vi "statsCalcWithWrite.vi"() -> ()   [LabVIEW 2014]
uses:
  <vilib>/gmath/statdist.llb/Normal Random.vi
  <userlib>/StatsCalculatorLabView/StatsCalculatorLabView.lvlib
  <vilib>/gmath/NI_Gmath.lvlib
  <vilib>/Analysis/NI_AALBase.lvlib
panel:
  in  "Output\nFilename":string="statsSummary.txt"
  out "VI Name":string
  out "Gaussian Distribution":T1(graph)
  out "Error State":errorcluster
  out "Standard Deviation":dbl(knob) scale=0.0..10.0
  out "Mean":dbl(knob) scale=0.0..10.0
  out "Sum":dbl(knob) scale=0.0..10.0
  in  "True\nStandard Deviation":dbl(knob)=0.5 scale=0.5..2.0
  in  "True Mean":dbl(knob) scale=-5.0..5.0
  in  "Number of Values":i32(knob)=50 scale=100.0..1000.0
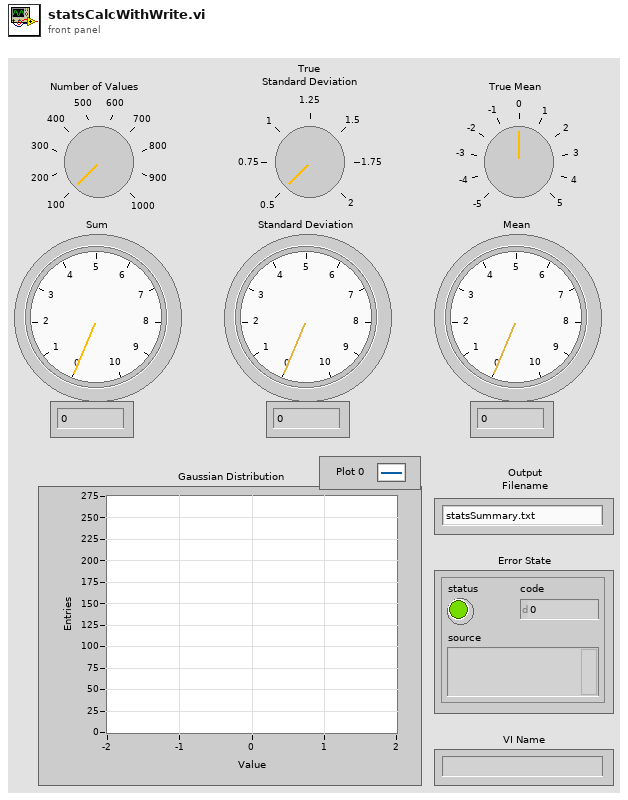
[diagram p1: front panel]
types:
  T1 = cluster{"X Values":dbl[], "Histogram: h(x)":i32[]}
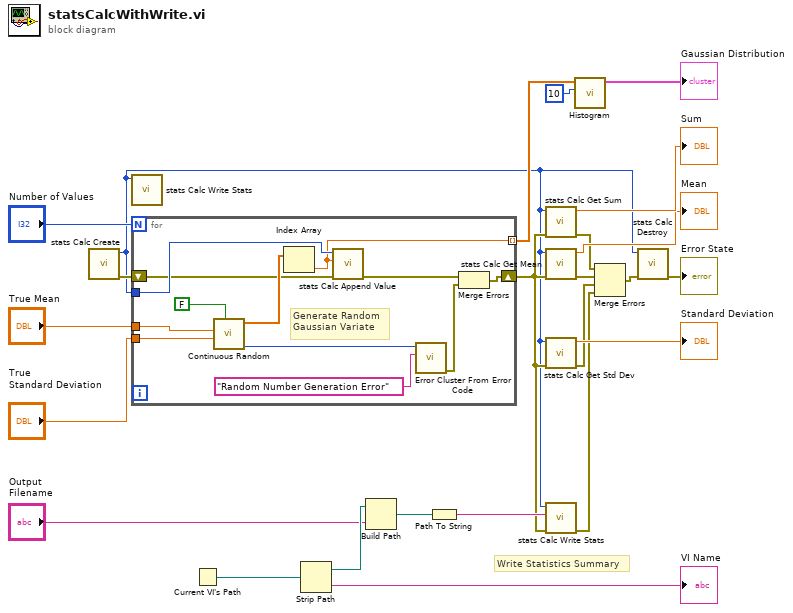
[diagram p0: block diagram]
diagram:
  # "Write Statistics Summary"
  n1 = call <userlib>:"stats Calc Create.vi"() -> ("error out"=w21:errorcluster, "function return"=w2:i32)  [unwired: 10 in]
  n2 = call <userlib>:"stats Calc Write Stats.vi"("handle"=w2) -> ()  [unwired: 10 in, 1 out]
  n3 = for {
    N: "Number of Values" -> [_]
    tunnel: w2 -> [w36]
    tunnel: "True\nStandard Deviation" -> [w35]
    tunnel: "True Mean" -> [w34]
    shift-right: [w26] -> w3
    shift-left: w21 -> [w29]
    tunnel: [w25] -> w12 mode=indexing
    # "Generate Random\nGaussian Variate"
    n4 = call-poly <vilib>:"Continuous Random.vi"("reset"=FALSE, "std"=w35, "mean"=w34) -> ("error"=w31:i32, "normal random data"=w32:dbl[])  [unwired: 7 in]
    n5 = Index Array(array=w32) -> (element=w25:dbl)  [unwired: 1 in]
    n6 = call <userlib>:"stats Calc Append Value.vi"("error in (no error)"=w29, "value"=w25, "handle"=w36) -> ("error out"=w27:errorcluster)  [unwired: 8 in]
    n7 = call <vilib>:"Error Cluster From Error Code.vi"("error message (\"\")"="Random Number Generation Error", "error code (0)"=w31) -> ("error out"=w28:errorcluster)  [unwired: 7 in]
    n8 = Merge Errors(w27, w28) -> (w26:errorcluster)
  }
  n9 = Current VI's Path() -> (path=w9:path)
  n10 = Strip Path(path=w9) -> (stripped path=w7:path, name=→"VI Name":string)
  n11 = Build Path(base path=w7, name or relative path="Output\nFilename") -> (appended path=w5:path)
  n12 = Path To String(path=w5) -> (string=w4:string)
  n13 = call <userlib>:"stats Calc Get Sum.vi"("error in (no error)"=w3, "handle"=w2) -> ("error out"=w17:errorcluster, "function return"=→"Sum":dbl)  [unwired: 8 in]
  n14 = call <userlib>:"stats Calc Get Mean.vi"("error in (no error)"=w3, "handle"=w2) -> ("error out"=w16:errorcluster, "function return"=→"Mean":dbl)  [unwired: 8 in]
  n15 = call <userlib>:"stats Calc Get Std Dev.vi"("error in (no error)"=w3, "handle"=w2) -> ("error out"=w15:errorcluster, "function return"=→"Standard Deviation":dbl)  [unwired: 8 in]
  n16 = call <userlib>:"stats Calc Write Stats.vi"("error in (no error)"=w3, "fileName"=w4, "handle"=w2) -> ("error out"=w1:errorcluster)  [unwired: 8 in]
  n17 = call <vilib>:"Histogram.vi"("intervals"=10, "X"=w12) -> ("Histogram Graph"=→"Gaussian Distribution":T1)  [unwired: 6 in, 3 out]
  n18 = Merge Errors(w17, w16, w15, w1) -> (w14:errorcluster)
  n19 = call <userlib>:"stats Calc Destroy.vi"("error in (no error)"=w14, "handle"=w2) -> ("error out"=→"Error State":errorcluster)  [unwired: 9 in]
